vi "Hybrid PS Read gateway.vi"() -> ()   [LabVIEW 2025]
doc: "Author: Scott Hannahs <sth@magnet.fsu.edu>\n\nThis software is licensed for use under the “MIT License\"\nCopyright (c) 2025 Scott Hannahs, sth@sth@magnet.sthnet.net\n\nPermission is hereby granted, free of charge, to any person obtaining a copy of this software and associated documentation files (the \"Software\"), to deal in the Software without restriction, including without limitation the rights to use, copy, modify, merge, publish, distribute, sublicense, and/or sell copies of the Software, and to permit persons to whom the Software is furnished to do so, subject to the following conditions: The above copyright notice and this permission notice shall be included in all copies or substantial portions of the Software.\n\nTHE SOFTWARE IS PROVIDED \"AS IS\", WITHOUT WARRANTY OF ANY KIND, EXPRESS OR IMPLIED, INCLUDING BUT NOT LIMITED TO THE WARRANTIES OF MERCHANTABILITY, FITNESS FOR A PARTICULAR PURPOSE AND NONINFRINGEMENT. IN NO EVENT SHALL THE AUTHORS OR COPYRIGHT HOLDERS BE LIABLE FOR ANY CLAIM, DAMAGES OR OTHER LIABILITY, WHETHER IN AN ACTION OF CONTRACT, TORT OR OTHERWISE, ARISING FROM, OUT OF OR IN CONNECTION WITH THE SOFTWARE OR THE USE OR OTHER DEALINGS IN THE SOFTWARE."
uses:
  Sub Controls/PS Status.ctl
  PS Comm Globals.vi
panel:
  out "Status":T1
  out "Max Slew [A/s]":dbl caption="Current [kA]" format="%.5f"
  out "Currents":cluster{"Current":dbl, "SC Current":dbl} {"SC Current" format="%.5f"; "Current" format="%.5f"}
  out "Max Current [kA]":dbl caption="Current [kA]" format="%.5f"
  out "Setpoint [kA]":dbl caption="Current [kA]" format="%.5f"
  in  "stop":bool
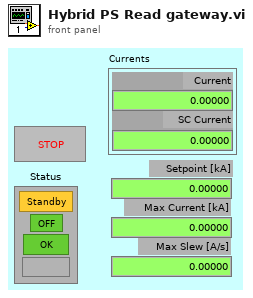
[diagram p1: front panel]
types:
  T1 = typedef "PS Status.ctl" = cluster{"PS On":bool, "PS Fault":bool, "Ramp Status":u16, "Cell Control":bool}
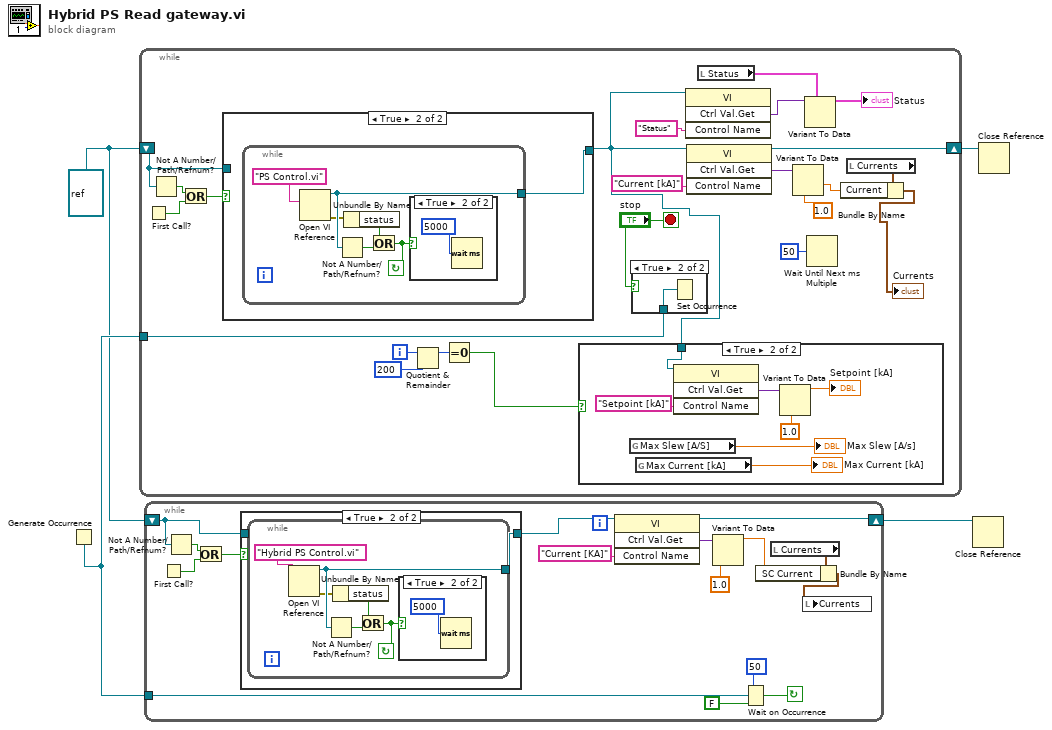
[diagram p0: block diagram]
diagram:
  w2 = refnum<vi> refnum
  n1 = Generate Occurrence() -> (w4:refnum<k4>)
  n2 = while {
    tunnel: w4 -> [w23]
    shift-right: [w17] -> w1
    shift-left: w2 -> [w18]
    i -> [w14]
    stop <- "stop" stop-if-true
    n3 = First Call?() -> (First Call?: T/F=w20:bool)
    n4 = Not A Number/Path/Refnum?(number/path/refnum=w18) -> (NaN/Path/Refnum?=w21:bool)
    n5 = Or(x=w21, y=w20) -> (x .or. y?=w19:bool)
    n6 = case shown="True" w19 {
      tunnel: [w35 w36] -> w9
      tunnel: w18 -> [w35 _]
      frame False {
      }
      frame True {
        n7 = while {
          tunnel: [w40] -> w36
          stop <- w37 continue-if-true
          n8 = Open VI Reference(vi path="PS Control.vi") -> (vi reference=w40:refnum<vi>, error out=w39:errorcluster)  [unwired: 5 in]
          n9 = Not A Number/Path/Refnum?(number/path/refnum=w40) -> (NaN/Path/Refnum?=w41:bool)
          n10 = Unbundle By Name(w39) -> ("status"=w38:bool)
          n11 = Or(x=w38, y=w41) -> (x .or. y?=w37:bool)
          n12 = case shown="True" w37 {
            frame False {
            }
            frame True {
              n13 = Wait (ms)(milliseconds to wait=u32 5000) -> ()  [unwired: 1 out]
            }
          }
        }
      }
    }
    n14 = Quotient & Remainder(x=w14, y=200) -> (x-y*floor(x/y)=w12:i32)  [unwired: 1 out]
    n15 = Equal To 0?(x=w12) -> (x = 0?=w11:bool)
    n16 = case shown="True" w11 {
      tunnel: w9 -> [_ w29]
      frame False {
      }
      frame True {
        n17 = global read "PS Comm Globals.vi" "Max Slew [A/S]"() -> (→"Max Slew [A/s]":dbl)
        n18 = global read "PS Comm Globals.vi" "Max Current [kA]"() -> (→"Max Current [kA]":dbl)
        n19 = invoke class="VI" method="Ctrl Val.Get"(reference=w29, "Control Name"="Setpoint [kA]") -> ("Get Control Value Variant"=w30:variant)  [unwired: 2 in, 3 out]
        n20 = Variant To Data(type=1.0, Variant=w30) -> (data=→"Setpoint [kA]":dbl)  [unwired: 1 in, 1 out]
      }
    }
    n21 = case shown="True" "stop" {
      tunnel: w23 -> [_ w44]
      frame False {
      }
      frame True {
        n22 = Set Occurrence(w44) -> ()
      }
    }
    n23 = invoke class="VI" method="Ctrl Val.Get"(reference=w9, "Control Name"="Status") -> ("Get Control Value Variant"=w7:variant)  [unwired: 2 in, 3 out]
    n24 = invoke class="VI" method="Ctrl Val.Get"(reference=w9, "Control Name"="Current [kA]") -> (reference out=w17:refnum<vi>, "Get Control Value Variant"=w25:variant)  [unwired: 2 in, 2 out]
    n25 = local read "Status"() -> (w5:T1)
    n26 = Variant To Data(type=1.0, Variant=w25) -> (data=w15:dbl)  [unwired: 1 in, 1 out]
    n27 = Variant To Data(type=w5, Variant=w7) -> (data=→"Status":T1)  [unwired: 1 in, 1 out]
    n28 = Wait Until Next ms Multiple(millisecond multiple=u32 50) -> ()  [unwired: 1 out]
    n29 = local read "Currents"() -> (w16:cluster{"Current":dbl, "SC Current":dbl})
    n30 = Bundle By Name(cluster=w16, "Current"=w15) -> (→"Currents":cluster{"Current":dbl, "SC Current":dbl})
  }
  n31 = while {
    tunnel: w4 -> [w56]
    shift-right: [w53] -> w3
    shift-left: w2 -> [w49]
    stop <- w57 continue-if-true
    n32 = First Call?() -> (First Call?: T/F=w52:bool)
    n33 = Not A Number/Path/Refnum?(number/path/refnum=w49) -> (NaN/Path/Refnum?=w51:bool)
    n34 = Or(x=w51, y=w52) -> (x .or. y?=w50:bool)
    n35 = case shown="True" w50 {
      tunnel: [w61 w62] -> w48
      tunnel: w49 -> [w61 _]
      frame False {
      }
      frame True {
        n36 = while {
          tunnel: [w66] -> w62
          stop <- w63 continue-if-true
          n37 = Open VI Reference(vi path="Hybrid PS Control.vi") -> (vi reference=w66:refnum<vi>, error out=w65:errorcluster)  [unwired: 5 in]
          n38 = Not A Number/Path/Refnum?(number/path/refnum=w66) -> (NaN/Path/Refnum?=w67:bool)
          n39 = Unbundle By Name(w65) -> ("status"=w64:bool)
          n40 = Or(x=w64, y=w67) -> (x .or. y?=w63:bool)
          n41 = case shown="True" w63 {
            frame False {
            }
            frame True {
              n42 = Wait (ms)(milliseconds to wait=u32 5000) -> ()  [unwired: 1 out]
            }
          }
        }
      }
    }
    n43 = invoke class="VI" method="Ctrl Val.Get"(reference=w48, "Control Name"="Current [KA]") -> (reference out=w53:refnum<vi>, "Get Control Value Variant"=w58:variant)  [unwired: 2 in, 2 out]
    n44 = Variant To Data(type=1.0, Variant=w58) -> (data=w47:dbl)  [unwired: 1 in, 1 out]
    n45 = Wait on Occurrence(1:FALSE ("ignore previous (T)"), 2:w56, 3:50 ("ms timeout (-1)")) -> (0:w57:bool)
    n46 = local read "Currents"() -> (w46:cluster{"Current":dbl, "SC Current":dbl})
    n47 = Bundle By Name(cluster=w46, "SC Current"=w47) -> (w45:cluster{"Current":dbl, "SC Current":dbl})
    n48 = local write "Currents"(w45) -> ()
  }
  n49 = Close Reference(reference=w3) -> ()  [unwired: 1 in, 1 out]
  n50 = Close Reference(reference=w1) -> ()  [unwired: 1 in, 1 out]
